vi "Get Process.vi"(8 "error in (no error)":errorcluster, 10 "Process Name":string, 11 "Application In":refnum<class "Application.lvclass">) -> (0 "error out":errorcluster, 2 "App Process":refnum<class "Process.lvclass">, 3 "Application Out":refnum<class "Application.lvclass">)   [LabVIEW 2020, in "Application.lvclass"]
doc: "Get a specific process by name. A good pattern for using this VI is to wrap it with a string constant fed into the Process Name input and cast the received process to the expected process class. This pattern makes changing the class or the name easy as there is only one this single location where it is specified.\nThe VI can return processes from nested applications using the qualified name of the process."
uses:
  Application.lvclass
  C:/git/astemes-triarc-framework/source/Framework/Process/Process.lvclass
  Process/Process.lvclass
  C:/git/astemes-triarc-framework/source/Framework/Logging/Logging.lvclass
  Application.lvclass/Application.ctl
  Process/Process.lvclass/Process.ctl
  Process/Protected/Messaging/Request Message.vi
  Private/Add Process to Map.vi
  <vilib>/AdvancedString/Delimited String to 1D String Array.vi
  Process/Protected/Messaging/Async Request Message.vi
  Process/Private/SubVIs/Handle Debug Data.vi
  Logging/Log Debug.vi
  <vilib>/AdvancedString/1D String Array to Delimited String.vi
  <vilib>/Utility/High Resolution Relative Seconds.vi
  Synchronous Request Callback/Synchronous Request Callback.lvclass
  C:/git/astemes-triarc-framework/source/Framework/Callback/Callback.lvclass
  Process/Public/Read Name.vi
  <vilib>/Utility/error.llb/Error Cluster From Error Code.vi
  Synchronous Request Callback/Create.vi
  Process/Private/SubVIs/Wait for Response Message.vi
  Callback/Callback.lvclass
  Logging/Logging.lvclass
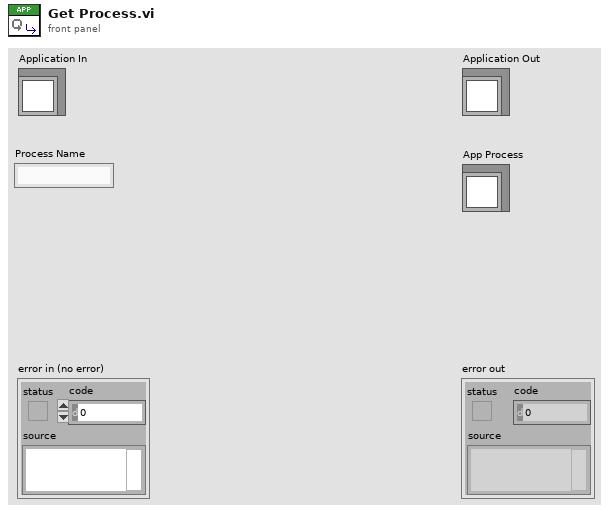
[diagram p1: front panel]
types:
  T1 = typedef "Process.lvclass/API Mode.ctl" = enum16{"Send Message", "Handle Message"}
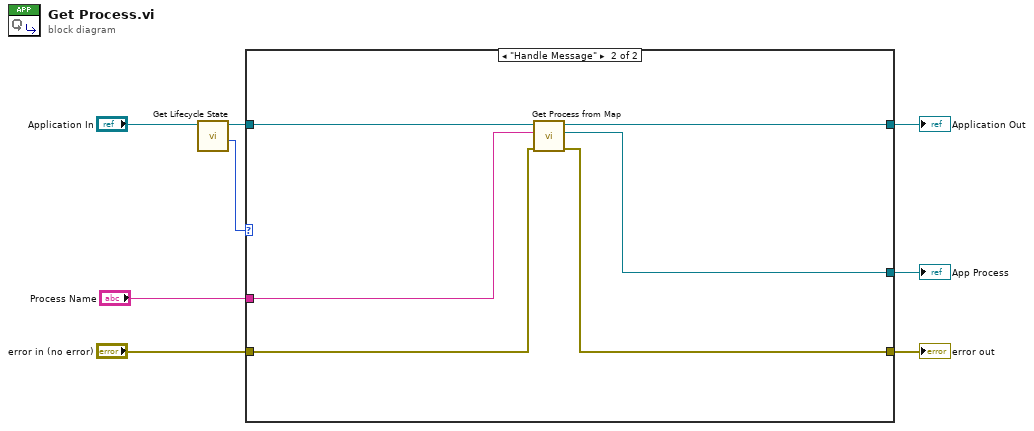
[diagram p0: block diagram]
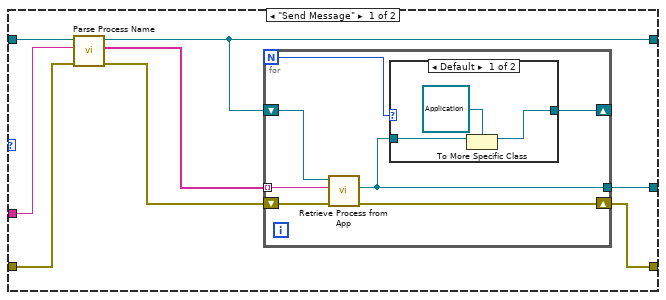
[diagram p2: hidden frame]
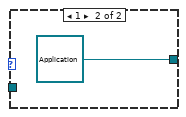
[diagram p3: hidden frame]
diagram:
  n1 = call "Get Lifecycle State.vi"("Process In"="Application In") -> ("API Mode"=w1:T1, "Process Out"=w2:refnum<class "Application.lvclass">)  [unwired: 7 in, 2 out]
  n2 = case shown="\"Handle Message\"" w1 {
    tunnel: [w16 w29] -> w8
    tunnel: [w15 w28] -> w7
    tunnel: "Process Name" -> [w14 w30]
    tunnel: "error in (no error)" -> [w12 w31]
    tunnel: [w10 w33] -> w3
    tunnel: w2 -> [w9 w32]
    frame "Send Message" {
      n3 = call "Parse Process Name.vi"("error in (no error)"=w12, "Process Name"=w14, "Application In"=w9) -> ("error out"=w11:errorcluster, "Array"=w13:string[], "Application Out"=w10:refnum<class "Application.lvclass">)  [unwired: 6 in]
      n4 = for {
        N -> [w17]
        tunnel: [w19] -> w16
        tunnel: w13 -> [w21] mode=indexing
        shift-right: [w18] -> _
        shift-left: w10 -> [w22]
        shift-right: [w23] -> w15
        shift-left: w11 -> [w20]
        n5 = call "Retrieve Process from App.vi"("error in (no error)"=w20, "String"=w21, "Application In"=w22) -> ("error out"=w23:errorcluster, "Process"=w19:refnum<class "Process.lvclass">)  [unwired: 6 in, 1 out]
        n6 = case shown="Default" w17 {
          tunnel: w19 -> [w26 _]
          tunnel: [w25 refnum<class "Application.lvclass"> refnum ("Application out")] -> w18
          frame Default {
            n7 = To More Specific Class(target class=refnum<class "Application.lvclass"> refnum ("Application out"), reference=w26) -> (specific class reference=w25:refnum<class "Application.lvclass">)  [unwired: 1 in, 1 out]
          }
          frame 1 {
          }
        }
      }
    }
    frame "Handle Message" {
      n8 = call "Get Process from Map.vi"("error in (no error)"=w31, "Process Name"=w30, "Application In"=w32) -> ("error out"=w28:errorcluster, "Process"=w29:refnum<class "Process.lvclass">, "Application Out"=w33:refnum<class "Application.lvclass">)  [unwired: 6 in]
    }
  }
  "error out" <- w7
  "Application Out" <- w3
  "App Process" <- w8
